vi "test.vi"() -> ()   [LabVIEW 2014]
panel:
  in  "stop":bool
  in  "buttons":T1
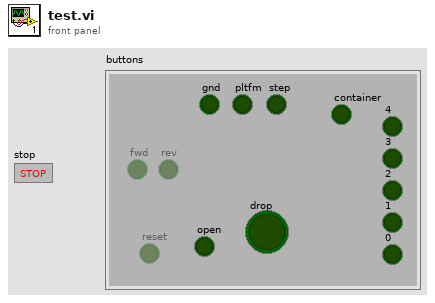
[diagram p1: front panel]
types:
  T1 = cluster{"0":bool, "1":bool, "2":bool, "3":bool, "4":bool, "container":bool, "step":bool, "pltfm":bool, "gnd":bool, "drop":bool, "fwd":bool, "rev":bool, "reset":bool, "open":bool}
  T2 = typedef "LEDPorts.ctl" = cluster{"Port":i16, "On Value":u8, "Off Value":u8}[][]
  T3 = cluster{"Port":i16, "On Value":u8, "Off Value":u8}
  T4 = cluster{"Port":i16, "On Value":u8, "Off Value":u8}[]
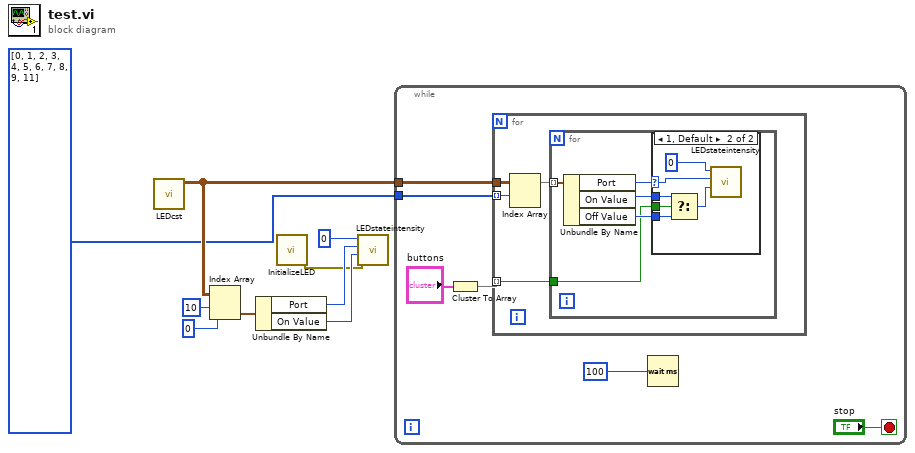
[diagram p0: block diagram]
diagram:
  n1 = call "LEDcst.vi"() -> ("Lights Values"=w2:T2)  [unwired: 11 in]
  n2 = Index Array(array=w2, index (row)=10, index (col)=0 ("disabled index (col)")) -> (element=w9:T3)
  n3 = Unbundle By Name(w9) -> ("Port"=w6:i16, "On Value"=w5:u8)
  n4 = call "InitializeLED.vi"() -> ("error out"=w4:errorcluster)  [unwired: 11 in]
  n5 = call "LEDstateintensity.vi"("error in (no error)"=w4, "intensity"=w5, "port"=w6, "Id"=i16 0) -> ()  [unwired: 5 in, 3 out]
  n6 = while {
    tunnel: w2 -> [w12]
    tunnel: i32[] [0, 1, 2, 3, 4, 5, 6, 7, 8, 9, 11] -> [w10]
    stop <- "stop" stop-if-true
    n7 = Cluster To Array(cluster="buttons") -> (array=w13:bool[])
    n8 = for {
      tunnel: w13 -> [w17] mode=indexing
      tunnel: w12 -> [w19]
      tunnel: w10 -> [w16] mode=indexing
      n9 = Index Array(array=w19, index (row)=w16) -> (element=w18:T4)  [unwired: 1 in]
      n10 = for {
        tunnel: w18 -> [w24] mode=indexing
        tunnel: w17 -> [w20]
        n11 = Unbundle By Name(w24) -> ("Port"=w23:i16, "On Value"=w22:u8, "Off Value"=w21:u8)
        n12 = case shown="1, Default" w23 {
          selector: w23 -> [_ w29]
          tunnel: w22 -> [_ w28]
          tunnel: w21 -> [_ w27]
          tunnel: w20 -> [_ w26]
          frame 0 {
          }
          frame 1, Default {
            n13 = Select(t=w28, s=w26, f=w27) -> (s? t:f=w25:u8)
            n14 = call "LEDstateintensity.vi"("intensity"=w25, "port"=w29, "Id"=i16 0) -> ()  [unwired: 6 in, 3 out]
          }
        }
      }
    }
    n15 = Wait (ms)(milliseconds to wait=u32 100) -> ()  [unwired: 1 out]
  }
